vi "Select Mask.vi"(6 "error in":errorcluster, 7 "Prompt":string="Select Left Mask", 8 "Read \nImage":T3(plugin-control)=refnum) -> (0 "error out":errorcluster, 1 "Cancelled":bool, 2 "ROI Descriptor Out":T1 {"Contours"."Type" items=["No Selection", "Point", "Line", "Rectangle", "Oval", "Polygon", "Freehand Region", "Annulus", "Unused2", "Unused3", "Broken Line", "Freehand Line", "Rotated Rectangle"]}, 3 "Masked \nImage":T3(plugin-control), 4 "Annulus":T2={"Center X"=982, "Center Y"=650, "Inner Radius"=309, "Outer Radius"=405, "Start Angle"=90.0, "End Angle"=180.0} {"End Angle" format="%.2f"; "Start Angle" format="%.2f"; "Center X" scale=0.0..1024.0}, 5 "mask":T3(plugin-control))   [LabVIEW 2013, in "Image Processing.lvlib"]
uses:
  Image Processing.lvlib
  <vilib>/vision/NI_Vision_Development_Module.lvlib
panel:
  in  "End Point":cluster{"X":i32, "Y":i32}
  in  "Start Point":cluster{"X":i32, "Y":i32}
  in  "Annulus Angles":cluster{"Start Angle":dbl, "End Angle":dbl}={"Start Angle"=0.0, "End Angle"=90.0}
  in  "Set Window Coordinates":cluster{"X Position":i32, "Y Position":i32}={"X Position"=0, "Y Position"=100}
  out "Window Coordinates":cluster{"X Position":i32, "Y Position":i32}={"X Position"=0, "Y Position"=100}
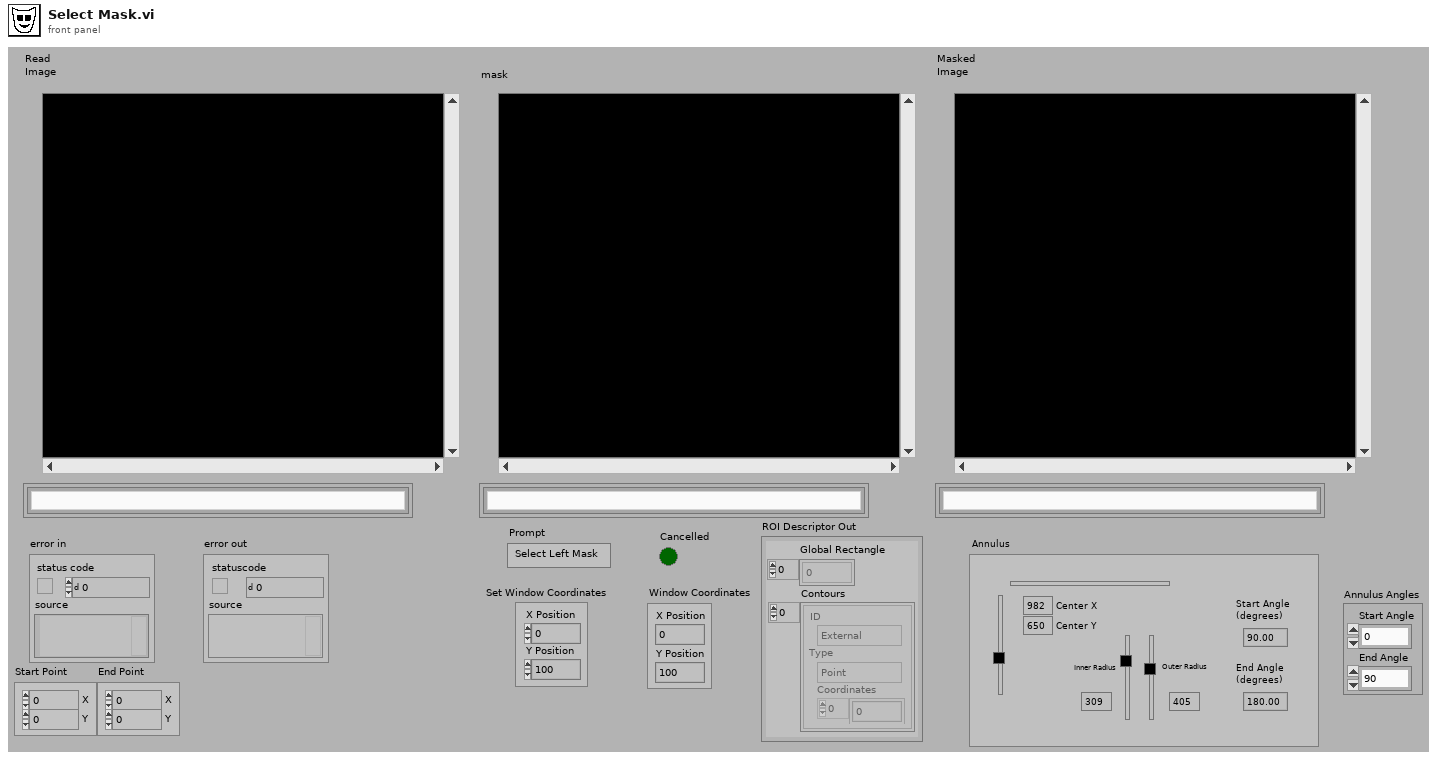
[diagram p1: front panel]
types:
  T1 = typedef "ROI Descriptor" = cluster{"Global Rectangle":i32[], "Contours":cluster{"ID":enum32{"External", "Internal"}, "Type":u32, "Coordinates":i32[]}[]}
  T2 = typedef "IMAQ Circle" = cluster{"Center X":i32, "Center Y":i32, "Inner Radius":i32, "Outer Radius":i32, "Start Angle":dbl, "End Angle":dbl}
  T3 = typedef "IMAQ Image.ctl" = refnum<image>
  T4 = enum32{"Gray", "Binary", "Gradient", "Rainbow", "Temperature"}
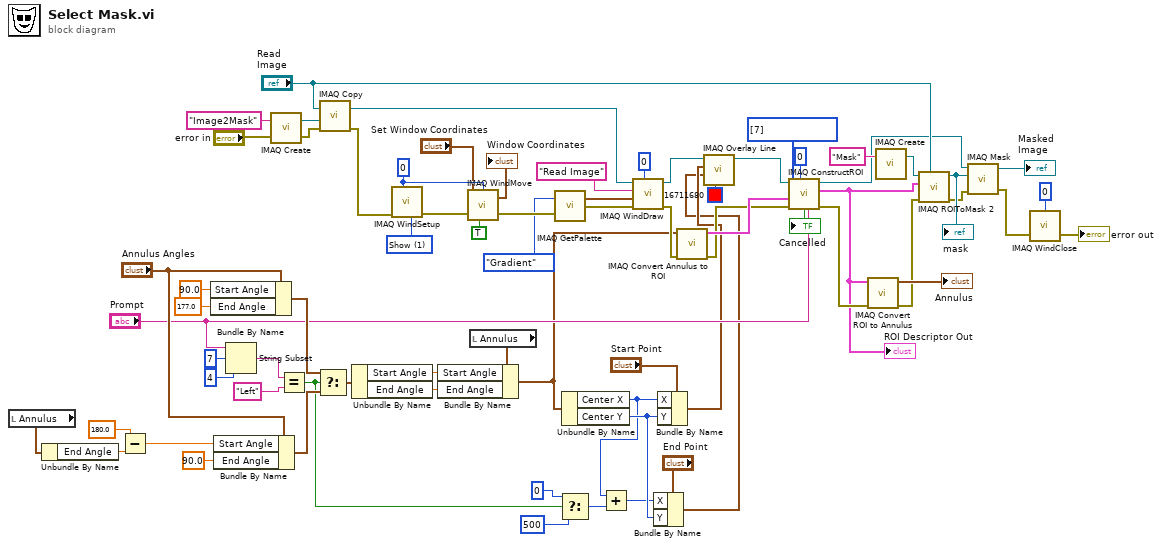
[diagram p0: block diagram]
diagram:
  w32 = u32[] [7] items=["No Selection", "Point", "Line", "Rectangle", "Oval", "Polygon", "Freehand Region", "Annulus", "Zoom", "Pan", "Broken Line", "Freehand Line", "Rotated Rectangle"] ("Tools")
  w64 = 1 items=["Hide", "Show", "No change"] ("Scrollbars (No change)")
  w60 = 0 ("Window Number (0...15)")
  n1 = local read "Annulus"() -> (w19:T2)
  n2 = Unbundle By Name(w19) -> ("End Angle"=w18:dbl)
  n3 = Subtract(x=180.0, y=w18) -> (x-y=w16:dbl)
  n4 = Bundle By Name(cluster="Annulus Angles", "Start Angle"=90.0, "End Angle"=177.0) -> (w42:cluster{"Start Angle":dbl, "End Angle":dbl})
  n5 = Bundle By Name(cluster="Annulus Angles", "Start Angle"=w16, "End Angle"=90.0) -> (w39:cluster{"Start Angle":dbl, "End Angle":dbl})
  n6 = String Subset(string="Prompt", offset (0)=7, length (rest)=4 ("length (rest)")) -> (substring=w45:string)
  n7 = call "IMAQ Create"("Image Name"="Image2Mask", "error in (no error)"="error in") -> ("New Image"=w56:T3, "error out"=w52:errorcluster)  [unwired: 3 in]
  n8 = Equal?(x=w45, y="Left") -> (x = y?=w7:bool)
  n9 = Select(t=w42, s=w7, f=w39) -> (s? t:f=w38:cluster{"Start Angle":dbl, "End Angle":dbl})
  n10 = call "IMAQ Copy"("error in (no error)"=w52, "Image Dst"=w56, "Image Src"="Read \nImage") -> ("error out"=w50:errorcluster, "Image Dst Out"=w54:T3)  [unwired: 3 in]
  n11 = Unbundle By Name(w38) -> ("Start Angle"=w37:dbl, "End Angle"=w36:dbl)
  n12 = call "IMAQ WindSetup"("Scrollbars (No change)"=w64, "Window Number (0...15)"=w60, "error in (no error)"=w50) -> ("error out"=w62:errorcluster)  [unwired: 8 in]
  n13 = call "IMAQ WindMove"("Window Number (0...15)"=w60, "Coordinates (screen)"="Set Window Coordinates", "Get/Set Status? (Set)"=TRUE, "error in (no error)"=w62) -> ("Coordinates (screen)"=→"Window Coordinates":cluster{"X Position":i32, "Y Position":i32}, "error out"=w59:errorcluster)  [unwired: 1 in]
  n14 = local read "Annulus"() -> (w49:T2)
  n15 = Bundle By Name(cluster=w49, "Start Angle"=w37, "End Angle"=w36) -> (w13:T2)
  n16 = call "IMAQ GetPalette"("Palette Number (gray)"=T4."Gradient", "error in (no error)"=w59) -> ("Color Palette"=w66:cluster{"Red":u8, "Green":u8, "Blue":u8}[], "error out"=w65:errorcluster)  [unwired: 3 in]
  n17 = Select(t=u16 0, s=w7, f=u16 500) -> (s? t:f=w5:u16)
  n18 = Unbundle By Name(w13) -> ("Center X"=w2:i32, "Center Y"=w9:i32)
  n19 = Add(x=w2, y=w5) -> (x+y=w4:i32)
  n20 = call "IMAQ WindDraw"("Window Number (0...15)"=0, "error in (no error)"=w65, "Color Palette"=w66, "Title"="Read Image", "Image"=w54) -> ("error out"=w35:errorcluster, "Image Out (duplicate)"=w15:T3)  [unwired: 1 in, 4 out]
  n21 = Bundle By Name(cluster="End Point", "X"=w4, "Y"=w9) -> (w1:cluster{"X":i32, "Y":i32})
  n22 = Bundle By Name(cluster="Start Point", "X"=w2, "Y"=w9) -> (w10:cluster{"X":i32, "Y":i32})
  n23 = call "IMAQ Convert Annulus to ROI"("error in (no error)"=w35, "Annulus"=w13) -> ("error out"=w30:errorcluster, "ROI Descriptor"=w31:T1)  [unwired: 7 in]
  n24 = call "IMAQ Overlay Line"("Color"=u32 16711680, "End Point"=w1, "Start Point"=w10, "Image"=w15) -> ("Image Out"=w14:T3)  [unwired: 6 in, 1 out]
  n25 = call "IMAQ ConstructROI"("Prompt"="Prompt", "Window Number (-1...15)"=0 ("Window Number (0...15)"), "error in (no error)"=w30, "ROI Descriptor In (None)"=w31, "Tools"=w32, "Image"=w14) -> ("error out"=w34:errorcluster, "Cancel"=→"Cancelled":bool, "ROI Descriptor Out"=w25:T1, "Image Out (duplicate)"=w28:T3)  [unwired: 2 in]
  "ROI Descriptor Out" <- w25
  n26 = call "IMAQ Convert ROI to Annulus"("error in (no error)"=w34, "ROI Descriptor"=w25) -> ("error out"=w24:errorcluster, "Annulus"=→"Annulus":T2)  [unwired: 7 in]
  n27 = call "IMAQ Create"("Image Name"="Mask") -> ("New Image"=w69:T3)  [unwired: 3 in, 2 out]
  n28 = call "IMAQ ROIToMask 2"("Image Model"="Read \nImage", "error in (no error)"=w24, "ROI Descriptor"=w25, "Image"=w69) -> ("error out"=w68:errorcluster, "Image Out"=w71:T3)  [unwired: 5 in, 1 out]
  "mask" <- w71
  n29 = call "IMAQ Mask"("error in (no error)"=w68, "Image Mask"=w71, "Image Src"=w28) -> ("error out"=w22:errorcluster, "Image Dst Out"=→"Masked \nImage":T3)  [unwired: 1 in, 1 out]
  n30 = call "IMAQ WindClose"("Window Number (0...15)"=0, "error in (no error)"=w22) -> ("error out"=→"error out":errorcluster)  [unwired: 4 in]
